vi "Comm String LastRead Message.vi"(8 "error in (no error)":errorcluster, 11 "niDTS Comm String in":refnum<class "niDTS Comm String.lvclass">) -> (0 "error out":errorcluster, 3 "niDTS Comm String out":refnum<class "niDTS Comm String.lvclass">)   [LabVIEW 2015, in "niDTS CommLib.lvlib" / "niDTS Comm String.lvclass"]
uses:
  niDTS Comm String.lvclass
  Framework/Logger/Includes/niDTS Logger INC Log Element Type.ctl
  Framework/Logger/Objects/BASE_class/niDTS Logger.lvclass
  Framework/niDTS Framework.lvlib
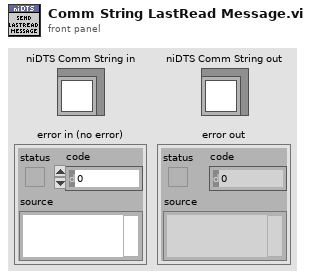
[diagram p1: front panel]
types:
  T1 = typedef "niDTS Framework.lvlib/niDTS Logger INC Log Element Type.ctl" = enum16{"Error", "Warning", "Information", "Debugging"}
  T2 = typedef "niDTS Framework.lvlib/niDTS Logger INC Handle.ctl" = refnum<data-value>
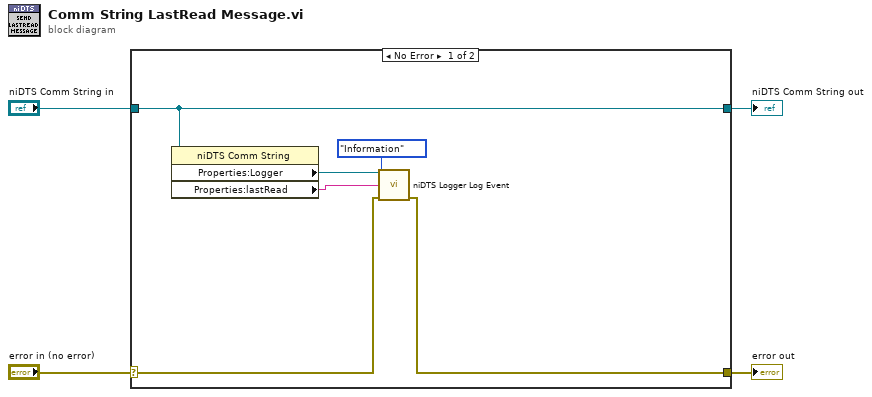
[diagram p0: block diagram]
diagram:
  n1 = case shown="No Error" "error in (no error)" {
    selector: "error in (no error)" -> [w6 w12]
    tunnel: [w5 w12] -> w3
    tunnel: [w10 w11] -> w1
    tunnel: "niDTS Comm String in" -> [w10 w11]
    frame No Error {
      n2 = property class="niDTS Comm String"(reference=w10) -> ("Properties:Logger"=w9:T2, "Properties:lastRead"=w7:string)  [unwired: 1 in, 2 out]
      n3 = call "niDTS Logger Log Event.vi"("Logger Handle"=w9, "Type"=niDTS_Logger_INC_Log_Element_Type."Information", "Description/Data"=w7, "error in (no error)"=w6) -> ("error out"=w5:errorcluster)  [unwired: 9 in, 2 out]
    }
    frame Error {
    }
  }
  "error out" <- w3
  "niDTS Comm String out" <- w1
